vi "Decimation DBL.vi"(9 "Decimation Array":dbl[](array[numeric]), 10 "Number of Bytes per Chunck (1000)":i32=1000, 11 "Raw Data":dbl[](array[numeric])) -> (3 "Decimation Data":dbl[](array[numeric]))   [LabVIEW 2020, in "Agilent 90000 Series.lvlib"]
doc: "Decimation on an DBL raw data array."
uses:
  Agilent 90000 Series.lvlib
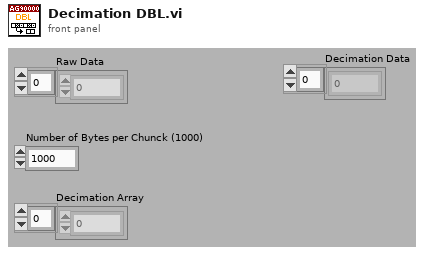
[diagram p1: front panel]
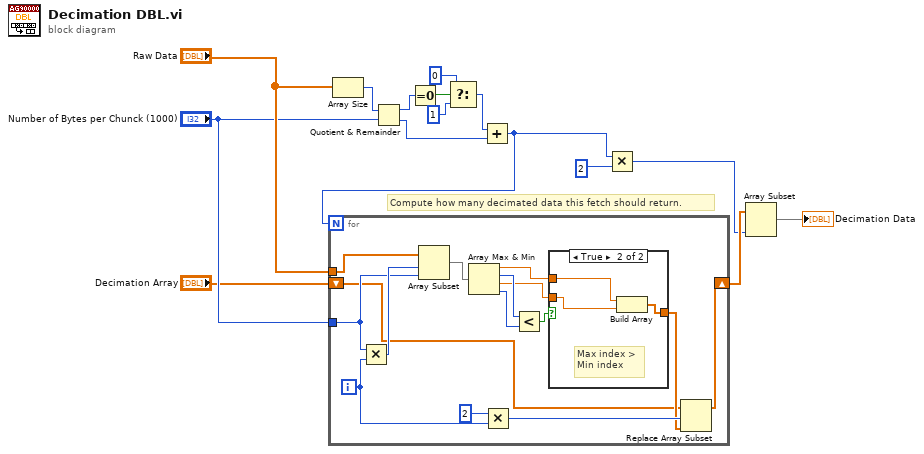
[diagram p0: block diagram]
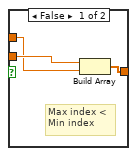
[diagram p2: hidden frame]
diagram:
  # "Compute how many decimated data this fetch should return."
  n1 = Array Size(array="Raw Data") -> (size(s)=w15:i32)
  n2 = Quotient & Remainder(x=w15, y="Number of Bytes per Chunck (1000)") -> (x-y*floor(x/y)=w12:i32, floor(x/y)=w13:i32)
  n3 = Equal To 0?(x=w12) -> (x = 0?=w11:bool)
  n4 = Select(t=0 ("y"), s=w11, f=1 ("y")) -> (s? t:f=w8:i32)
  n5 = Add(x=w8, y=w13) -> (x+y=w5:i32)
  n6 = for {
    N: w5 -> [_]
    tunnel: "Number of Bytes per Chunck (1000)" -> [w29]
    tunnel: "Raw Data" -> [w22]
    shift-right: [w21] -> w14
    shift-left: "Decimation Array" -> [w16]
    i -> [w20]
    n7 = Multiply(x=w29, y=w20) -> (x*y=w30:i32)
    n8 = Array Subset(array=w22, index=w30, length=w29) -> (w23:dbl[])
    n9 = Array Max & Min(array=w23) -> (max value=w25:dbl, max index (indices)=w28:i32, min value=w24:dbl, min index (indices)=w27:i32)
    n10 = Multiply(x=2, y=w20) -> (x*y=w18:i32)
    n11 = Less?(x=w28, y=w27) -> (x < y?=w26:bool)
    n12 = case shown="True" w26 {
      tunnel: w25 -> [w32 w36]
      tunnel: w24 -> [w33 w35]
      tunnel: [w31 w34] -> w17
      frame False {
        # "Max index <\nMin index"
        n13 = Build Array(w33, w32) -> (w31:dbl[])
      }
      frame True {
        # "Max index >\nMin index"
        n14 = Build Array(w36, w35) -> (w34:dbl[])
      }
    }
    n15 = Replace Array Subset(array=w16, new element=w17, index=w18) -> (w21:dbl[])
  }
  n16 = Multiply(x=w5, y=2) -> (x*y=w3:i32)
  n17 = Array Subset(array=w14, length=w3) -> (→"Decimation Data":dbl[])  [unwired: 1 in]
